vi "Dereference Glyph Record.vi"(8 "error in (no error)":errorcluster, 11 "glyph ref in":i64) -> (0 "error out":errorcluster, 2 "out":T1, 3 "glyph ref out":i64)   [LabVIEW 2023, in "Freetype Drawer.lvlib"]
uses:
  Freetype Drawer.lvlib
  Glyph Slot Rec.ctl
  FT Metrics RAW.ctl
  FT Bitmap.ctl
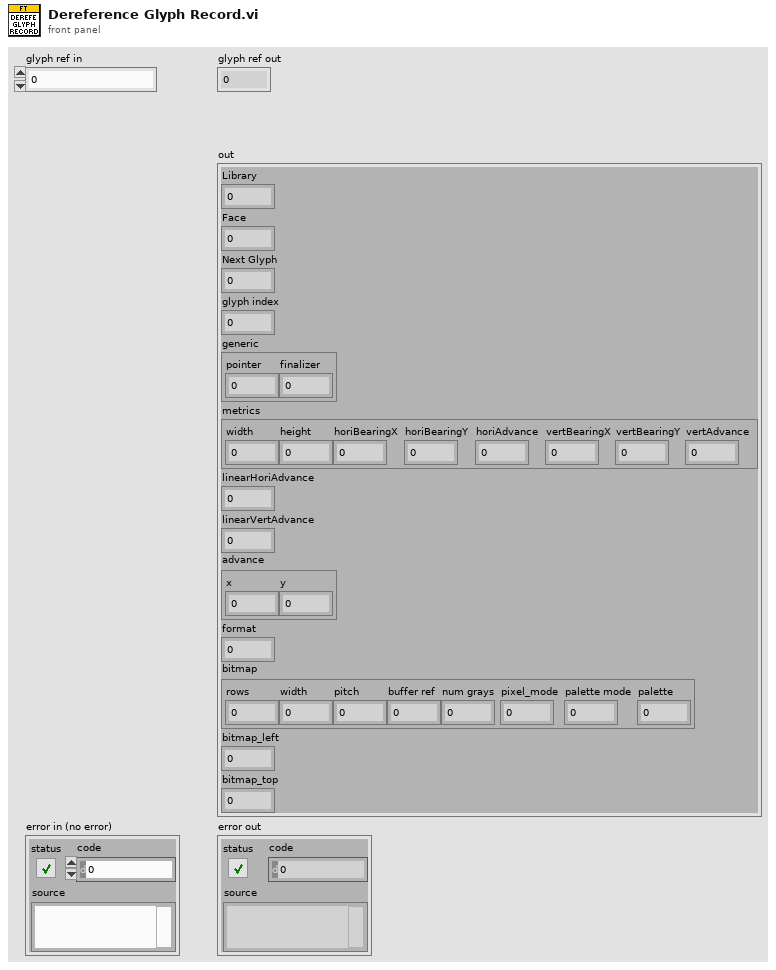
[diagram p1: front panel]
types:
  T1 = typedef "Freetype Drawer.lvlib/Glyph Slot Rec.ctl" = cluster{"Library":i64, "Face":i64, "Next Glyph":i64, "glyph index":u32, "generic":cluster{"pointer":i64, "finalizer":i64}, "metrics":T2, "linearHoriAdvance":i32, "linearVertAdvance":i32, "advance":cluster{"x":i32, "y":i32}, "format":i32, "bitmap":T3, "bitmap_left":i32, "bitmap_top":i32}
  T2 = typedef "Freetype Drawer.lvlib/FT Metrics RAW.ctl" = cluster{"width":i32, "height":i32, "horiBearingX":i32, "horiBearingY":i32, "horiAdvance":i32, "vertBearingX":i32, "vertBearingY":i32, "vertAdvance":i32}
  T3 = typedef "Freetype Drawer.lvlib/FT Bitmap.ctl" = cluster{"rows":u32, "width":u32, "pitch":i32, "buffer ref":i64, "num grays":i16, "pixel_mode":u8, "palette mode":u8, "palette":i64}
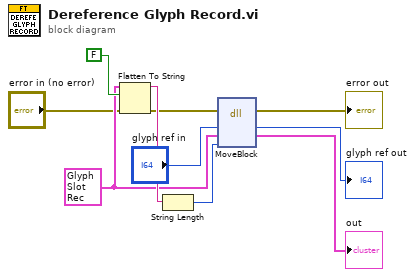
[diagram p0: block diagram]
diagram:
  w7 = T1 {"Library"=0, "Face"=0, "Next Glyph"=0, "glyph index"=0, "generic"={"pointer"=0, "finalizer"=0}, "metrics"={"width"=0, "height"=0, "horiBearingX"=0, "horiBearingY"=0, "horiAdvance"=0, "vertBearingX"=0, "vertBearingY"=0, "vertAdvance"=0}, "linearHoriAdvance"=0, "linearVertAdvance"=0, "advance"={"x"=0, "y"=0}, "format"=0, "bitmap"={"rows"=0, "width"=0, "pitch"=0, "buffer ref"=0, "num grays"=0, "pixel_mode"=0, "palette mode"=0, "palette"=0}, "bitmap_left"=0, "bitmap_top"=0} ("Glyph")
  n1 = Flatten To String(anything=w7, prepend array or string size? (T)=FALSE, error in (no error)="error in (no error)") -> (data string=w9:string, error out=w3:errorcluster)  [unwired: 1 in, 1 out]
  n2 = String Length(string=w9) -> (length=w1:i32)
  n3 = dll-call lib="LabVIEW" fn="MoveBlock"(error in=w3, "in"="glyph ref in", "out"=w7, "size"=w1) -> (error out=→"error out":errorcluster, "in"=→"glyph ref out":i64, "out"=→"out":T1)  [unwired: 4 in, 1 out]
